vi "LUCS001RT_GPS_RS232_Receiver.vi"(6 "FPGA VI Reference In":T3, 8 "error in":errorcluster, 11 "SinchronizationReferences":T1) -> (0 "error out":errorcluster, 2 "RX ArrayReady":bool, 3 "GPS.TX.Message":u8[](array[numeric]) format="%02x")   [LabVIEW 2020]
uses:
  <vilib>/rvi/interface/nirviMethod/nirviMethod.xnode
  SourceCode_Host/FPGA Bitfiles/LUCS001h.lvproj_FPGA Target 1_LUCS001FPGA_Main.vi.lvbit
  SourceCodeFPGA/LUCS001FPGA_Main.vi
  <vilib>/rvi/errors/niLvFpgaMergeErrorWithErrorCode.vi
  cRIO Projects LV8.5/UAV/TypeDefs.llb/UMV_SinchronisationReferences.ctl
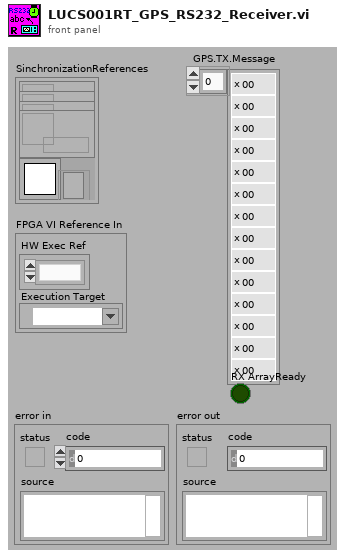
[diagram p1: front panel]
types:
  T1 = typedef "UMV_SinchronisationReferences.ctl" = cluster{"Notifier:LocalStop":refnum<notifier>, "Notifier:GlobalStop":refnum<notifier>, "RS232write":refnum<queue>, "RS232read":refnum<queue>, "RS232writeSynch":T2, "occurrence":refnum<k4>}
  T2 = typedef "Semaphore RefNum" = refnum<k1>
  T3 = cluster{"HW Exec Ref":refnum<k1>, "Execution Target":refnum<visa-resource-name>}
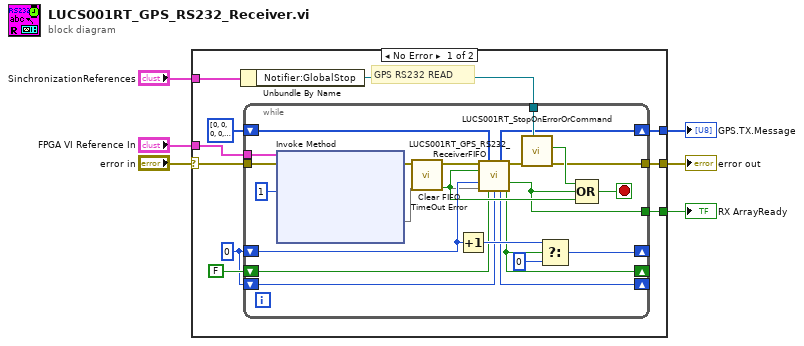
[diagram p0: block diagram]
diagram:
  n1 = case shown="No Error" "error in" {
    selector: "error in" -> [w13 w40]
    tunnel: [w12 w40] -> w4
    tunnel: "SinchronizationReferences" -> [w16 _]
    tunnel: "FPGA VI Reference In" -> [w14 _]
    tunnel: [w9 _] -> w6
    tunnel: [w7 _] -> w1
    frame No Error {
      w8 = 0 ("Number of Elements")
      # "GPS RS232 READ"
      n2 = Unbundle By Name(w16) -> ("Notifier:GlobalStop"=w15:refnum<notifier>)
      n3 = while {
        tunnel: w15 -> [w39]
        tunnel: w14 -> [w35]
        tunnel: w13 -> [w36]
        tunnel: [w37] -> w12
        shift-right: [w25] -> w9
        shift-left: u8[] [0, 0, 0, 0, 0, 0, 0, 0, 0, 0, 0, 0, 0, 0, 0, 0, 0, 0, 0, 0, 0, 0, 0, 0, 0, 0, 0, 0, 0, 0, 0, 0, 0, 0, 0, 0, 0, 0, 0, 0, 0, 0, 0, 0, 0, 0, 0, 0, 0, 0, 0, 0, 0, 0, 0, 0, 0, 0, 0, 0, 0, 0, 0, 0, 0, 0, 0, 0, 0, 0, 0, 0, 0, 0, 0, 0, 0, 0, 0, 0, 0, 0, 0, 0, 0, 0, 0, 0, 0, 0, 0, 0, 0, 0, 0, 0, 0, 0, 0, 0] ("CmpsTX.Message 2") -> [w26]
        shift-right: [w21] -> _
        shift-left: FALSE ("UpdateStateOut") -> [w22]
        shift-right: [w30] -> _
        shift-left: w8 -> [w24]
        shift-right: [w18] -> _
        shift-left: w8 -> [w19]
        tunnel: [w17] -> w7
        stop <- w29 stop-if-true
        n4 = xnode "Invoke Method"("FPGA VI Reference In"=w35, "error in"=w36, "Number of Elements"=u32 1) -> ("error out"=w33:errorcluster, "Data"=w20)  [unwired: 1 in, 2 out]
        n5 = call "Clear FIFO TimeOut Error.vi"("error in (no error)"=w33) -> ("TimedOut"=w23:bool, "error out"=w28:errorcluster)  [unwired: 9 in]
        n6 = Increment(x=w24) -> (x+1=w31:i32)
        n7 = call "LUCS001RT_GPS_RS232_ReceiverFIFO.vi"("error in"=w28, "RxArrayIn"=w26, "TimedOut"=w23, "CurrentLoopIndex"=w24, "FIFODataIn"=w20, "UpdateStateIn"=w22, "MarkIndexIn"=w19) -> ("RxArrayOut"=w25:u8[], "error out"=w27:errorcluster, "DataReady"=w17:bool, "MarkIndexOut"=w18:i32, "UpdateStateOut"=w21:bool)  [unwired: 4 in]
        n8 = call "LUCS001RT_StopOnErrorOrCommand.vi"("STOP"=w39, "error in (no error)"=w27) -> ("error out"=w37:errorcluster, "STOP_Out"=w38:bool)  [unwired: 8 in]
        n9 = Select(t=w31, s=w21, f=0 ("Number of Elements")) -> (s? t:f=w30:i32)
        n10 = Compound Arithmetic op=OR(w38, w17, w23) -> (w29:bool)
      }
    }
    frame Error {
    }
  }
  "GPS.TX.Message" <- w6
  "error out" <- w4
  "RX ArrayReady" <- w1
